vi "__init__.vi"(8 "error in (no error)":errorcluster, 11 "self in":refnum<class "AttrAlias.lvclass">) -> (0 "error out":errorcluster, 3 "self out":refnum<class "AttrAlias.lvclass">)   [LabVIEW 2020, in "mlir.lvlib" / "AttrAlias.lvclass"]
uses:
  AttrAlias.lvclass
  AttrAlias.lvclass/AttrAlias.ctl
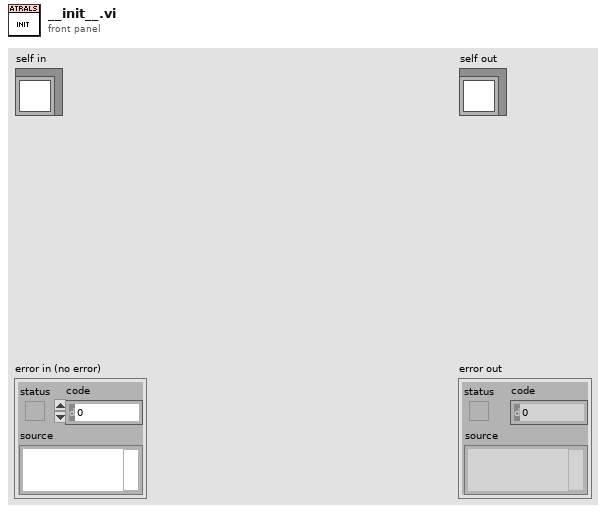
[diagram p1: front panel]
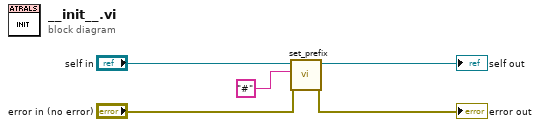
[diagram p0: block diagram]
diagram:
  n1 = call-dynamic "set_prefix.vi"("error in (no error)"="error in (no error)", "_prefix_"="#", "self in"="self in") -> ("error out"=→"error out":errorcluster, "self out"=→"self out":refnum<class "AttrAlias.lvclass">)  [unwired: 7 in]
